vi "Thread.vi"(8 "Error in":errorcluster caption="Error in (no error)", 11 "NUM":i32) -> (0 "Error out":errorcluster)   [LabVIEW 2020]
uses:
  <userlib>/_NEVSTOP/GlobalStop/_gStop.vi
  <userlib>/_NEVSTOP/GlobalStop/GSTOP.lvlib
panel:
  in  "stop":bool
  out "indicator":i32
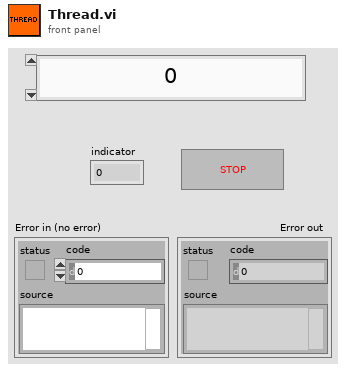
[diagram p1: front panel]
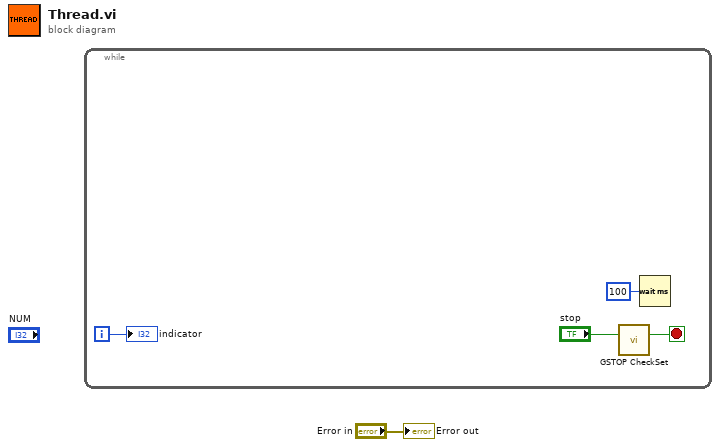
[diagram p0: block diagram]
diagram:
  n1 = while {
    i -> [w3]
    stop <- w2 stop-if-true
    n2 = call <userlib>:"GSTOP CheckSet.vi"("stop value"="stop") -> ("stop"=w2:bool)  [unwired: 13 in, 1 out]
    n3 = Wait (ms)(milliseconds to wait=u32 100) -> ()  [unwired: 1 out]
    "indicator" <- w3
  }
  "Error out" <- "Error in"
